vi "Read Plugin Runtime.vi"(8 "error in (no error)":errorcluster, 11 "Data Sharing Plugin in":refnum<class "Plugin.lvclass">) -> (0 "error out":errorcluster, 2 "Data Sharing Plugin Runtime":refnum<class "Plugin Runtime.lvclass">, 3 "Data Sharing Plugin out":refnum<class "Plugin.lvclass">)   [LabVIEW 2016, in "Plugin.lvclass"]
uses:
  Plugin.lvclass
  Plugin Runtime/Plugin Runtime.lvclass
  Plugin.lvclass/Plugin.ctl
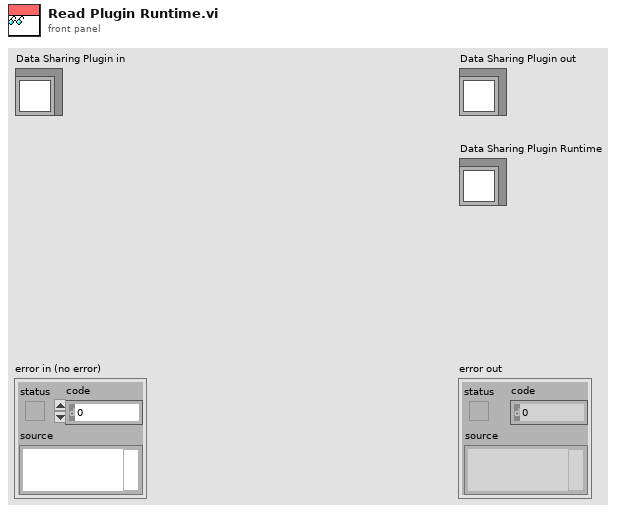
[diagram p1: front panel]
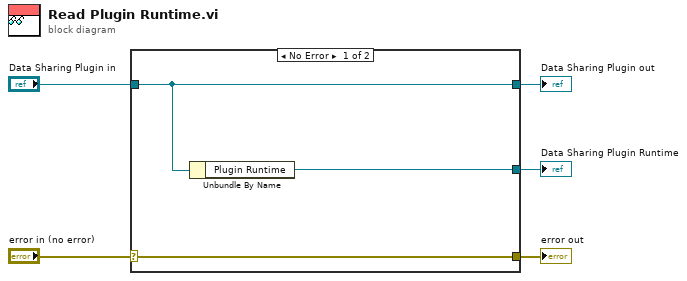
[diagram p0: block diagram]
diagram:
  n1 = case shown="No Error" "error in (no error)" {
    selector: "error in (no error)" -> [w8 w9]
    tunnel: [w8 w9] -> w4
    tunnel: [w7 w10] -> w2
    tunnel: "Data Sharing Plugin in" -> [w7 w10]
    tunnel: [w6 _] -> w1
    frame No Error {
      n2 = Unbundle By Name(w7) -> ("Plugin Runtime"=w6:refnum<class "Plugin Runtime.lvclass">)
    }
    frame Error {
    }
  }
  "error out" <- w4
  "Data Sharing Plugin out" <- w2
  "Data Sharing Plugin Runtime" <- w1
